vi "R_W_PLC Signal.vi"(8 "error in (no error)":errorcluster caption="错误输入（无错误）", 9 "PLC信号量设定":string[][](table), 10 "DO":T1, 11 "TCP In":refnum<k5>) -> (0 "error out":errorcluster caption="错误输出", 2 "DI":cluster{"孔径启动信号":bool, "铜片启动信号":bool}, 3 "TCP Out":refnum<k5>)   [LabVIEW 2017]
panel:
  out "连接的字符串 3":string
  out "trimmed string":string caption="删减后字符串"
  out "x = y?":bool
  out "布尔":bool
  out "连接的字符串 OK":string
  # "WRS MR30108 5 0 0 0 0 0"
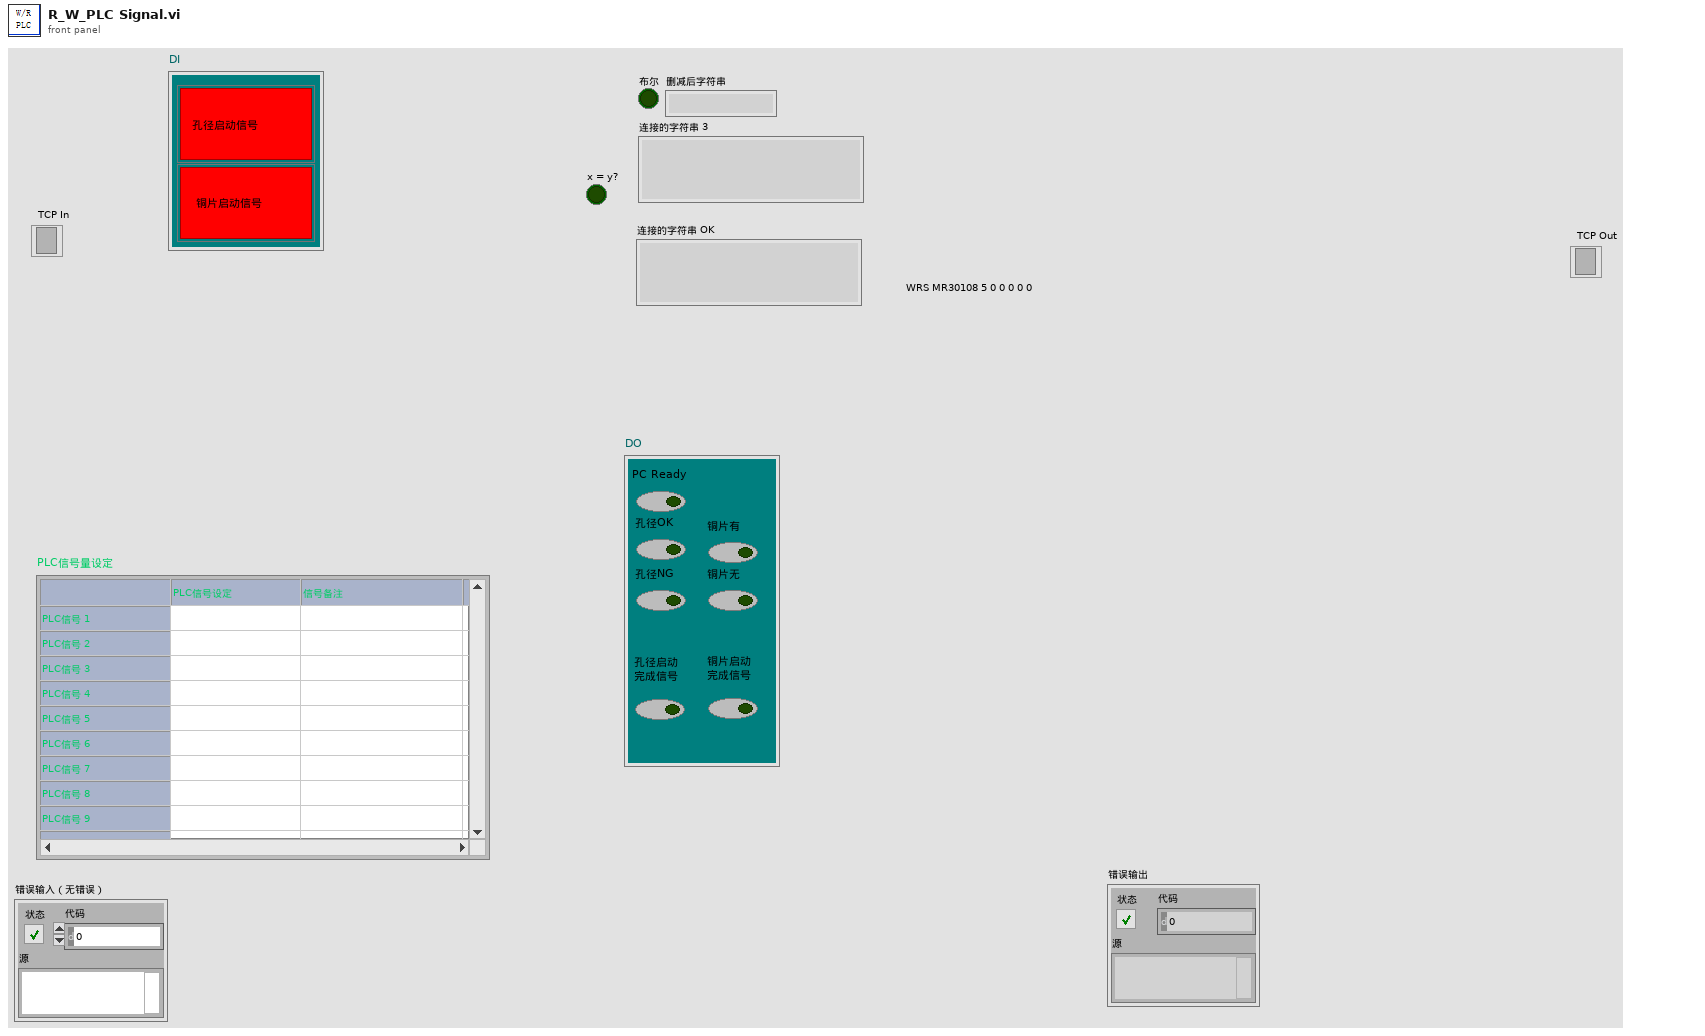
[diagram p1: front panel]
types:
  T1 = cluster{"PC Ready":bool, "孔径OK":bool, "孔径NG":bool, "铜片有":bool, "铜片无":bool, "孔径启动\n完成信号":bool, "铜片启动\n完成信号":bool}
  T2 = enum16{"Standard", "Buffered", "CRLF", "Immediate"}
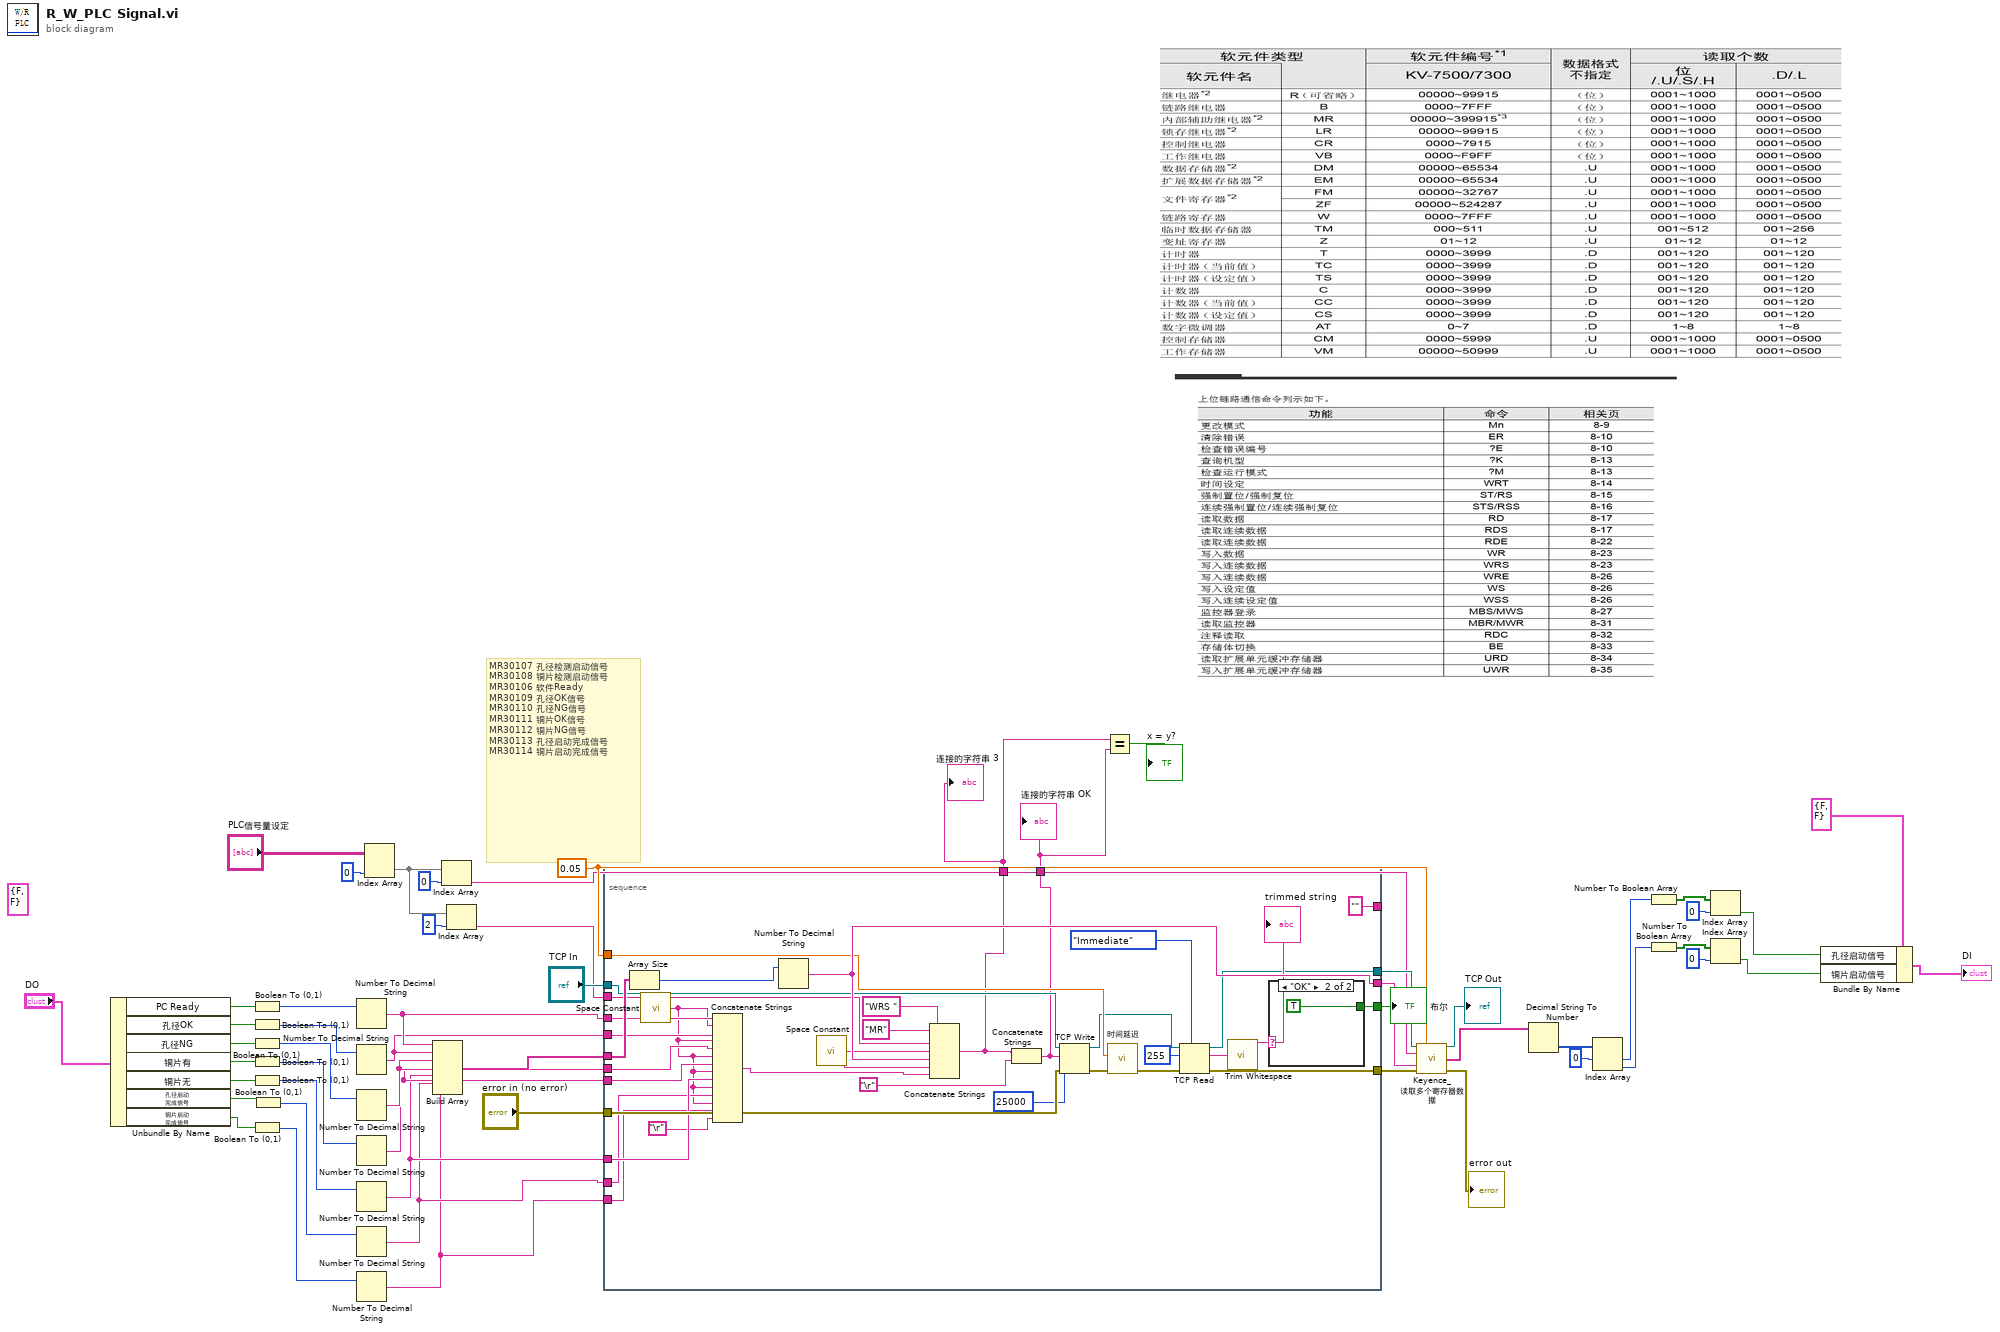
[diagram p0: block diagram]
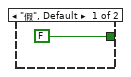
[diagram p2: hidden frame]
diagram:
  (unwired) cluster{"孔径启动信号":bool, "铜片启动信号":bool} {"孔径启动信号"=FALSE, "铜片启动信号"=FALSE} ("DI")
  w38 = 0.05 ("Delay Time (s)")
  # "MR30107\t孔径检测启动信号\nMR30108\t铜片检测启动信号\nMR30106\t软件Ready\nMR30109\t孔径OK信号\nMR30110\t孔径NG信号\nMR30111\t铜片OK信号\nMR30112\t铜片NG信号\nMR30113\t孔径启动完成信号\nMR30114\t铜片启动完成信号"
  n1 = Unbundle By Name("DO") -> ("PC Ready"=w51:bool, "孔径OK"=w50:bool, "孔径NG"=w49:bool, "铜片有"=w27:bool, "铜片无"=w26:bool, "孔径启动\n完成信号"=w6:bool, "铜片启动\n完成信号"=w5:bool)
  n2 = Boolean To (0,1)(Boolean=w51) -> (0, 1=w48:i16)
  n3 = Boolean To (0,1)(Boolean=w50) -> (0, 1=w47:i16)
  n4 = Boolean To (0,1)(Boolean=w49) -> (0, 1=w46:i16)
  n5 = Boolean To (0,1)(Boolean=w27) -> (0, 1=w25:i16)
  n6 = Boolean To (0,1)(Boolean=w26) -> (0, 1=w24:i16)
  n7 = Boolean To (0,1)(Boolean=w5) -> (0, 1=w3:i16)
  n8 = Boolean To (0,1)(Boolean=w6) -> (0, 1=w4:i16)
  n9 = Number To Decimal String(number=w48) -> (decimal integer string=w11:string)  [unwired: 1 in]
  n10 = Number To Decimal String(number=w47) -> (decimal integer string=w10:string)  [unwired: 1 in]
  n11 = Number To Decimal String(number=w46) -> (decimal integer string=w9:string)  [unwired: 1 in]
  n12 = Number To Decimal String(number=w25) -> (decimal integer string=w8:string)  [unwired: 1 in]
  n13 = Number To Decimal String(number=w24) -> (decimal integer string=w7:string)  [unwired: 1 in]
  n14 = Number To Decimal String(number=w4) -> (decimal integer string=w2:string)  [unwired: 1 in]
  n15 = Number To Decimal String(number=w3) -> (decimal integer string=w1:string)  [unwired: 1 in]
  n16 = Index Array(array="PLC信号量设定", index (col)=0 ("禁用的索引 (列)")) -> (element=w18:string[])  [unwired: 1 in]
  n17 = Build Array(w11, w10, w9, w8, w7, w2, w1) -> (w45:string[])
  n18 = Index Array(array=w18, index=0 ("索引")) -> (element=w17:string)
  n19 = Index Array(array=w18, index=2 ("索引")) -> (element=w16:string)
  n20 = stacked-sequence {
    tunnel: "TCP In" -> [w78]
    tunnel: w38 -> [w81]
    tunnel: [w85] -> w43
    tunnel: w16 -> [w84]
    tunnel: ["" ("数据输出")] -> _
    tunnel: [w90] -> w39
    tunnel: w45 -> [w89]
    tunnel: [w88] -> w15
    tunnel: "error in (no error)" -> [w79]
    tunnel: [w80] -> w41
    tunnel: [w68] -> w14
    tunnel: [w59] -> w12
    tunnel: w11 -> [w66]
    tunnel: w10 -> [w65]
    tunnel: w9 -> [w64]
    tunnel: w8 -> [w63]
    tunnel: w7 -> [w62]
    tunnel: w2 -> [w58]
    tunnel: w1 -> [w56]
    frame #0 {
      n21 = Array Size(array=w89) -> (size(s)=w75:i32)
      n22 = call <vilib>:"Space Constant.vi"() -> ("String"=w57:string)
      n23 = Concatenate Strings(w66, w57, w65, w57, w64, w57, w63, w57, w62, w57, w58, w57, w56, "\r") -> (w61:string)
      n24 = Number To Decimal String(number=w75) -> (decimal integer string=w90:string)  [unwired: 1 in]
      n25 = call <vilib>:"Space Constant.vi"() -> ("String"=w67:string)
      n26 = Concatenate Strings("WRS ", "MR" ("字符串"), w84, w67, w90, w67, w61) -> (w59:string)
      n27 = Concatenate Strings(w59, "\r") -> (w68:string)
      n28 = TCP Write(connection ID=w78, data in=w68, error in (no error)=w79, 9:25000 ("超时毫秒(25000)")) -> (connection ID out=w71:refnum<k5>, error out=w72:errorcluster)  [unwired: 1 out]
      n29 = call "时间延迟"("error in (no error)"=w72, "Delay Time (s)"=w81) -> ("error out"=w73:errorcluster)  [unwired: 9 in]
      n30 = TCP Read(connection ID=w71, bytes to read=255 ("读取的字节"), error in (no error)=w73, 7:T2."Immediate" ("模式（标准）")) -> (connection ID out=w85:refnum<k5>, data out=w86:string, error out=w80:errorcluster)  [unwired: 1 in]
      n31 = call <vilib>:"Trim Whitespace.vi"("string"=w86) -> ("trimmed string"=w87:string)  [unwired: 1 in]
      "trimmed string" <- w87
      n32 = case shown="\"OK\"" w87 {
        tunnel: [FALSE TRUE] -> w88
        frame "假", Default {
        }
        frame "OK" {
        }
      }
    }
  }
  "连接的字符串 OK" <- w14
  "布尔" <- w15
  "连接的字符串 3" <- w12
  n33 = Equal?(x=w12, y=w14) -> (x = y?=→"x = y?":bool)
  n34 = call "Keyence_读取多个寄存器数据.vi"("Keyence ID In"=w43, "Delay Time (s)"=w38, "起始软元件编号"=w17, "读取个数"=w39, "错误输入（无错误）"=w41) -> ("Keyence ID Out"=→"TCP Out":refnum<k5>, "结果数组"=w37:string[], "错误输出"=→"error out":errorcluster)  [unwired: 7 in, 1 out]
  n35 = Decimal String To Number(string=w37) -> (number=w36:i32[])  [unwired: 2 in, 1 out]
  n36 = Index Array(array=w36, index #1=0 ("索引")) -> (element #1=w34:i32, element #2=w23:i32)  [unwired: 1 in]
  n37 = Number To Boolean Array(number=w34) -> (Boolean array=w33:bool[])
  n38 = Number To Boolean Array(number=w23) -> (Boolean array=w29:bool[])
  n39 = Index Array(array=w33, index=0 ("索引")) -> (element=w31:bool)
  n40 = Index Array(array=w29, index=0 ("索引")) -> (element=w28:bool)
  n41 = Bundle By Name(cluster=cluster{"孔径启动信号":bool, "铜片启动信号":bool} {"孔径启动信号"=FALSE, "铜片启动信号"=FALSE} ("DI"), "孔径启动信号"=w31, "铜片启动信号"=w28) -> (→"DI":cluster{"孔径启动信号":bool, "铜片启动信号":bool})
